vi "Peak Hold.vi"(0 "real spectrum":dbl[](array[numeric]) format="%.2f", 1 "reset averaging":bool=TRUE) -> (2 "peak spectrum":dbl[](array[numeric]) format="%.2f", 3 "averages completed":dbl format="%.2f", 4 "error out":errorcluster)   [LabVIEW 2017]
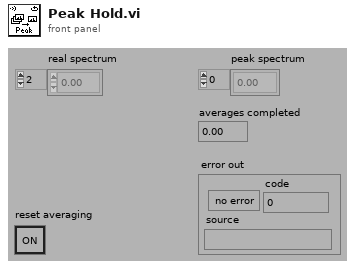
[diagram p1: front panel]
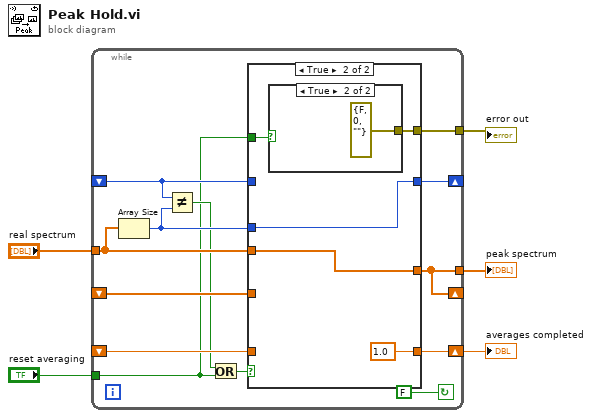
[diagram p0: block diagram]
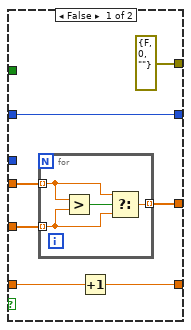
[diagram p2: hidden frame]
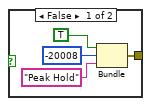
[diagram p3: hidden frame]
diagram:
  n1 = while {
    tunnel: [w8] -> w1
    shift-left: _ -> [w11]
    shift-right: [w13] -> _
    tunnel: "real spectrum" -> [w14]
    shift-left: _ -> [w16]
    shift-right: [w17] -> w2
    shift-left: _ -> [w15]
    shift-right: [w18] -> _
    tunnel: [w18] -> w3
    tunnel: "reset averaging" -> [w7]
    stop <- FALSE continue-if-true
    n2 = Array Size(array=w14) -> (size(s)=w12:i32)
    n3 = Not Equal?(x=w11, y=w12) -> (x != y?=w9:bool)
    n4 = Or(x=w9, y=w7) -> (x .or. y?=w10:bool)
    n5 = case shown="True" w10 {
      tunnel: [w21 w33] -> w18
      tunnel: [w24 1.0] -> w17
      tunnel: w16 -> [w25 _]
      tunnel: w15 -> [w22 _]
      tunnel: w14 -> [w23 w33]
      tunnel: w12 -> [_ w32]
      tunnel: w11 -> [w20 _]
      tunnel: [w20 w32] -> w13
      tunnel: [errorcluster {FALSE, 0, ""} w30] -> w8
      tunnel: w7 -> [_ w31]
      frame False {
        n6 = for {
          tunnel: w23 -> [w28] mode=indexing
          tunnel: w22 -> [w27] mode=indexing
          tunnel: [w26] -> w21 mode=indexing
          n7 = Greater?(x=w28, y=w27) -> (0:w29:bool)
          n8 = Select(t=w28, s=w29, f=w27) -> (s? t:f=w26:dbl)
        }
        n9 = Increment(x=w25) -> (x+1=w24:dbl)
      }
      frame True {
        n10 = case shown="True" w31 {
          tunnel: [w35 errorcluster {FALSE, 0, ""}] -> w30
          frame False {
            n11 = Bundle(TRUE, -20008, "Peak Hold") -> (w35:errorcluster)  [unwired: 1 in]
          }
          frame True {
          }
        }
      }
    }
  }
  "peak spectrum" <- w3
  "averages completed" <- w2
  "error out" <- w1
